vi "ExecuteListDecode.vi"(0 "Payload":string) -> (1 "Presence Vector":u8, 2 "Speed":dbl, 3 "Element UID":u16)   [LabVIEW 2009]
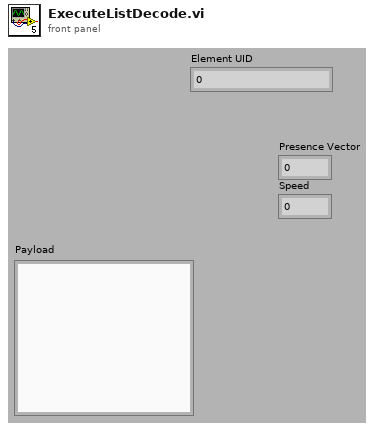
[diagram p1: front panel]
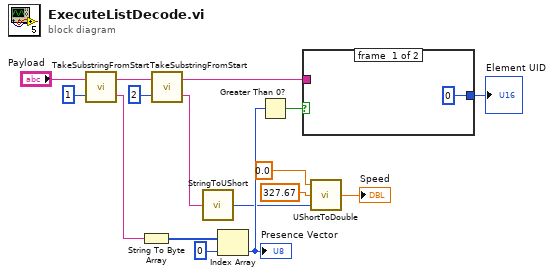
[diagram p0: block diagram]
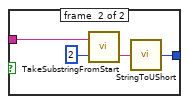
[diagram p2: hidden frame]
diagram:
  n1 = call "TakeSubstringFromStart.vi"("offset"=1, "string"="Payload") -> ("string before offset"=w14:string, "string after offset"=w10:string)
  n2 = String To Byte Array(string=w14) -> (unsigned byte array=w13:u8[])
  n3 = call "TakeSubstringFromStart.vi"("offset"=2, "string"=w10) -> ("string before offset"=w9:string, "string after offset"=w6:string)
  n4 = call "StringToUShort.vi"("string"=w9) -> ("UShort"=w4:u16)
  n5 = Index Array(array=w13, index=0) -> (element=w8:u8)
  "Presence Vector" <- w8
  n6 = Greater Than 0?(x=w8) -> (x > 0?=w7:bool)
  n7 = case shown="True" w7 {
    tunnel: w6 -> [_ w20]
    tunnel: [u16 0 ("UShort") w18] -> w5
    frame #0 {
    }
    frame #1 {
      n8 = call "TakeSubstringFromStart.vi"("offset"=2, "string"=w20) -> ("string before offset"=w19:string)  [unwired: 1 out]
      n9 = call "StringToUShort.vi"("string"=w19) -> ("UShort"=w18:u16)
    }
  }
  "Element UID" <- w5
  n10 = call "UShortToDouble.vi"("Value"=w4, "Max"=327.67, "Min"=0.0) -> ("Number"=→"Speed":dbl)
